vi "Check refnum if its IA CD.vi"(8 "Error In":errorcluster, 11 "Refnum In":T1 format="%.0x") -> (0 "Error Out":errorcluster, 2 "Is Instrument Addon?":bool, 3 "Refnum Out":u64)   [LabVIEW 2018, in "Instrument Addon Scripting API.lvlib"]
doc: "Verifies if the provided Refnum is an Instrument Addon Custom Device\n\nInput: \nRefnum In: represent the reference number which about to be compared agains the Instrument Addon GUID\n\nOutput: \nRefnum Out: represents the reference number provided as input\nIs Instrument Addon?: boolean value which indicates if the provided refnum references an Instrument Addon Custom Device"
uses:
  Instrument Addon Scripting API.lvlib
  <vilib>/NI Veristand/Custom Device API/Custom Device Item Ref.ctl
  Addon/Addon Shared/SubVIs/Constants.vi
  <vilib>/Utility/error.llb/Error Cluster From Error Code.vi
  <vilib>/ErrorRing/Error Ring.xnode
  <vilib>/NI/NI VeriStand Advanced SysDef API/SysDef API/Advanced System Definition.lvlib
  Addon/Addon Shared/Instrument Addon Shared.lvlib
  <vilib>/NI Veristand/Custom Device API/Custom Device API.lvlib
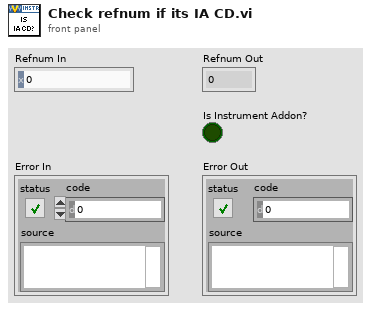
[diagram p1: front panel]
types:
  T1 = typedef "Custom Device API.lvlib/Custom Device Item Ref.ctl" = u64
  T2 = typedef "Advanced System Definition.lvlib/TreeItem.Info.ctl" = cluster{"Name":string, "Description":string, "GUID":string, "Is Channel":bool, "Channel":T3, "Is Waveform":bool, "Waveform":T5}
  T3 = typedef "Custom Device API.lvlib/Custom Device Channel.ctl" = cluster{"Type":T4, "Units":string, "Default Value":dbl, "Faultable":bool, "Scalable":bool}
  T4 = typedef "Custom Device API.lvlib/Custom Device Channel Type.ctl" = enum16{"Input", "Output"}
  T5 = typedef "Custom Device API.lvlib/Custom Device Waveform.ctl" = cluster{"Data Type":T6, "Units":string}
  T6 = typedef "Custom Device API.lvlib/Custom Device Waveform DataType.ctl" = enum16{"Double", "Complex Double"}
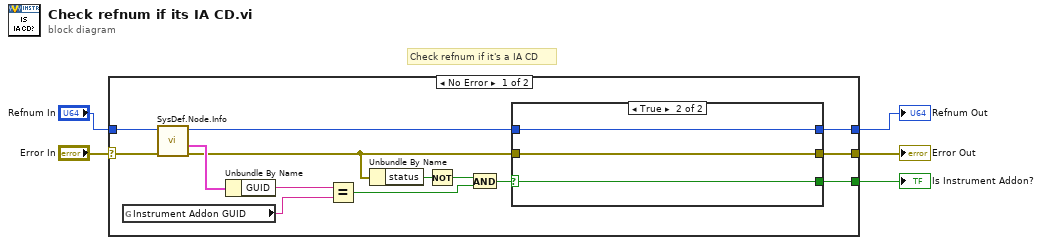
[diagram p0: block diagram]
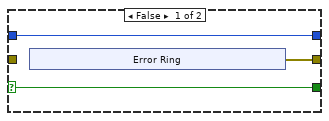
[diagram p2: hidden frame]
diagram:
  # "Check refnum if it's a IA CD"
  n1 = case shown="No Error" "Error In" {
    selector: "Error In" -> [w15 w31]
    tunnel: [w14 w31] -> w5
    tunnel: [w12 w32] -> w4
    tunnel: "Refnum In" -> [w16 w32]
    tunnel: [w11 _] -> w2
    frame No Error {
      n2 = global read "Constants.vi" "Instrument Addon GUID"() -> (w19:string)
      n3 = call <vilib>:"SysDef.Node.Info.vi"("error in (no error)"=w15, "nodeID"=w16) -> ("error out"=w6:errorcluster, "Item Info"=w17:T2, "nodeID out"=w13:u64)  [unwired: 6 in, 1 out]
      n4 = Unbundle By Name(w17) -> ("GUID"=w18:string)
      n5 = Equal?(x=w18, y=w19) -> (x = y?=w10:bool)
      n6 = Unbundle By Name(w6) -> ("status"=w9:bool)
      n7 = Not(x=w9) -> (.not. x?=w8:bool)
      n8 = And(x=w8, y=w10) -> (x .and. y?=w7:bool)
      n9 = case shown="True" w7 {
        selector: w7 -> [w20 w29]
        tunnel: [w21 w28] -> w14
        tunnel: w13 -> [w22 w30]
        tunnel: [w22 w30] -> w12
        tunnel: [w20 w29] -> w11
        tunnel: w6 -> [_ w28]
        frame False {
          n10 = xnode "Error Ring"() -> ("error out"=w21:errorcluster)
        }
        frame True {
        }
      }
    }
    frame Error {
    }
  }
  "Error Out" <- w5
  "Refnum Out" <- w4
  "Is Instrument Addon?" <- w2
